vi "FT10_Auto Next Power Operation.vi"(10 "Power Level in":T2, 11 "Power Reading":dbl) -> (3 "Auto Tester - Next Power Operation":T1)   [LabVIEW 2015]
uses:
  Controls/Control_Semi-Auto Power Level.ctl
  Controls/Control_Auto - Next Power Operation.ctl
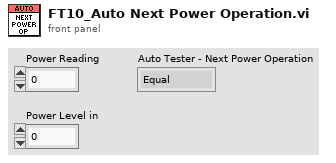
[diagram p1: front panel]
types:
  T1 = typedef "Control_Auto - Next Power Operation.ctl" = enum16{"Equal", "Power Down", "Power Up"}
  T2 = typedef "Control_Semi-Auto Power Level.ctl" = dbl
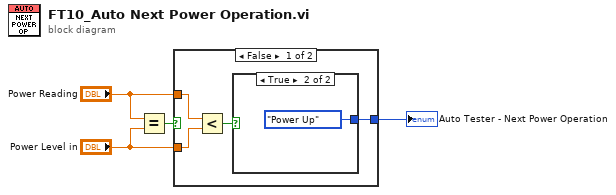
[diagram p0: block diagram]
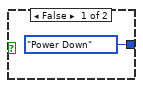
[diagram p2: hidden frame]
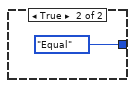
[diagram p3: hidden frame]
diagram:
  n1 = Equal?(x="Power Reading", y="Power Level in") -> (x = y?=w1:bool)
  n2 = case shown="False" w1 {
    tunnel: "Power Reading" -> [w7 _]
    tunnel: "Power Level in" -> [w6 _]
    tunnel: [w5 Control_Auto_-_Next_Power_Operation."Equal"] -> w4
    frame False {
      n3 = Less?(x=w7, y=w6) -> (x < y?=w8:bool)
      n4 = case shown="True" w8 {
        tunnel: [Control_Auto_-_Next_Power_Operation."Power Down" Control_Auto_-_Next_Power_Operation."Power Up"] -> w5
        frame False {
        }
        frame True {
        }
      }
    }
    frame True {
    }
  }
  "Auto Tester - Next Power Operation" <- w4
